vi "定点周期设置.vi"(11 "TimingControl 输入":refnum<class "TimingControl.lvclass">) -> (3 "TimingControl 输出":refnum<class "TimingControl.lvclass">)   [LabVIEW 2016, in "TimingControl.lvlib" / "TimingControl.lvclass"]
uses:
  TimingControl.lvclass
  TimingControl.lvclass/TimingControl.ctl
  <vilib>/Utility/miscctls.llb/LVPointTypeDef.ctl
panel:
  out "时间标识":timestamp format="%<%x %X>T"
  in  "每月启动":T1
  in  "每周启动":T2
  out "测试状态.结束时间":timestamp caption="结束时间" format="%<%y/%m/%d %H:%M:%S>T"
  out "测试状态.启动次数":dbl caption="启动次数"
  out "测试状态.启动时间":timestamp caption="启动时间" format="%<%y/%m/%d %H:%M:%S>T"
  in  "测量参数":T3 items=["氨氮"]
  in  "保存":bool
  in  "退出":bool
  in  "批量设置":bool
  out "周期模式选择卡":enum32{"选项卡 1", "选项卡 2"}(tab)
  in  "定点周期":T4
  in  "间隔启动":T6
  in  "周期模式":T7
  # "分钟"
  # "次"
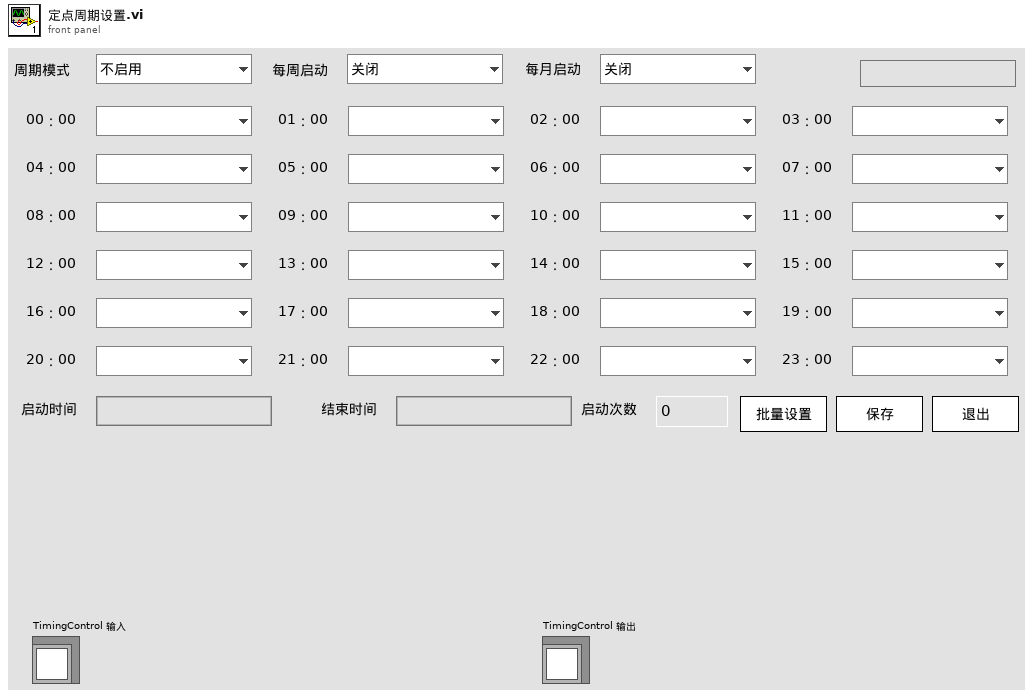
[diagram p1: front panel]
types:
  T1 = typedef "TimingControl.lvlib/TimingControl.lvclass/每月启动.ctl" = enum16{"关闭", "1号", "2号", "3号", "4号", "5号", "6号", "7号", "8号", "9号", "10号", "11号", "12号", "13号", "14号", "15号", "16号", "17号", "18号", "19号", "20号", "21号", "22号", "23号", "24号", "25号", "26号", "27号", "28号", "29号", "30号", "31号"}
  T2 = typedef "TimingControl.lvlib/TimingControl.lvclass/每周启动.ctl" = enum16{"关闭", "周日", "周一", "周二", "周三", "周四", "周五", "周六"}
  T3 = typedef "TimingControl.lvlib/TimingControl.lvclass/测量参数.ctl" = u16
  T4 = typedef "TimingControl.lvlib/TimingControl.lvclass/定点周期设置.ctl" = cluster{"启动命令":T5, "启动命令 2":T5, "启动命令 3":T5, "启动命令 4":T5, "启动命令 5":T5, "启动命令 6":T5, "启动命令 7":T5, "启动命令 8":T5, "启动命令 9":T5, "启动命令 10":T5, "启动命令 11":T5, "启动命令 12":T5, "启动命令 13":T5, "启动命令 14":T5, "启动命令 15":T5, "启动命令 16":T5, "启动命令 17":T5, "启动命令 18":T5, "启动命令 19":T5, "启动命令 20":T5, "启动命令 21":T5, "启动命令 22":T5, "启动命令 23":T5, "启动命令 24":T5}
  T5 = typedef "TimingControl.lvlib/TimingControl.lvclass/启动命令选择.ctl" = enum16{"", "水样测试", "标样核查", "零点核查", "跨度核查", "空白测试", "平行样测试", "加标回收", "空白校准", "标样校准", "初始化(清洗)"}
  T6 = typedef "TimingControl.lvlib/TimingControl.lvclass/间隔启动设置.ctl" = cluster{"启动命令":T5, "启动间隔":dbl, "启动次数":i32}
  T7 = typedef "TimingControl.lvlib/TimingControl.lvclass/周期模式设置.ctl" = enum16{"不启用", "定点模式", "间隔模式"}
  T8 = typedef "LVPointTypeDef.ctl" = cluster{"Horizontal":i16, "Vertical":i16}
  T9 = cluster{"启动时间":timestamp, "结束时间":timestamp, "启动次数":dbl}
  T10 = typedef "TimingControl.lvlib/TimingControl.lvclass/State Data.ctl" = cluster{"仪器时间":timestamp, "仪器运行状态":bool, "配置文件路径":path, "测量参数":u16, "测试状态":cluster{"启动时间":timestamp, "结束时间":timestamp, "启动次数":i32}, "配置信息":T11}
  T11 = typedef "TimingControl.lvlib/TimingControl.lvclass/配置信息.ctl" = cluster{"每周启动":T2, "每月启动":T1, "周期模式":T7, "测量参数":T3, "定点周期":T4, "间隔启动":T6, "配置时间":timestamp}
  T12 = cluster{"启动时间":timestamp, "结束时间":timestamp, "启动次数":i32}
  T13 = typedef "周期设置.lvlib/周期模式设置.ctl" = enum16{"不启用", "定点模式", "间隔模式"}
  T14 = typedef "LVDateTimeRec.ctl" = cluster{"秒数的小数部分":dbl, "秒":i32, "分":i32, "时":i32, "日":i32, "月":i32, "年":i32, "天数（周）":i32, "天数（年）":i32, "DST":i32}
  T15 = cluster{"每周启动":T2, "每月启动":T1, "周期模式":T7, "测量参数":T3, "定点周期":T4, cluster{"启动命令":T5, "启动间隔":dbl, "启动次数":i32}, "time stamp":timestamp}
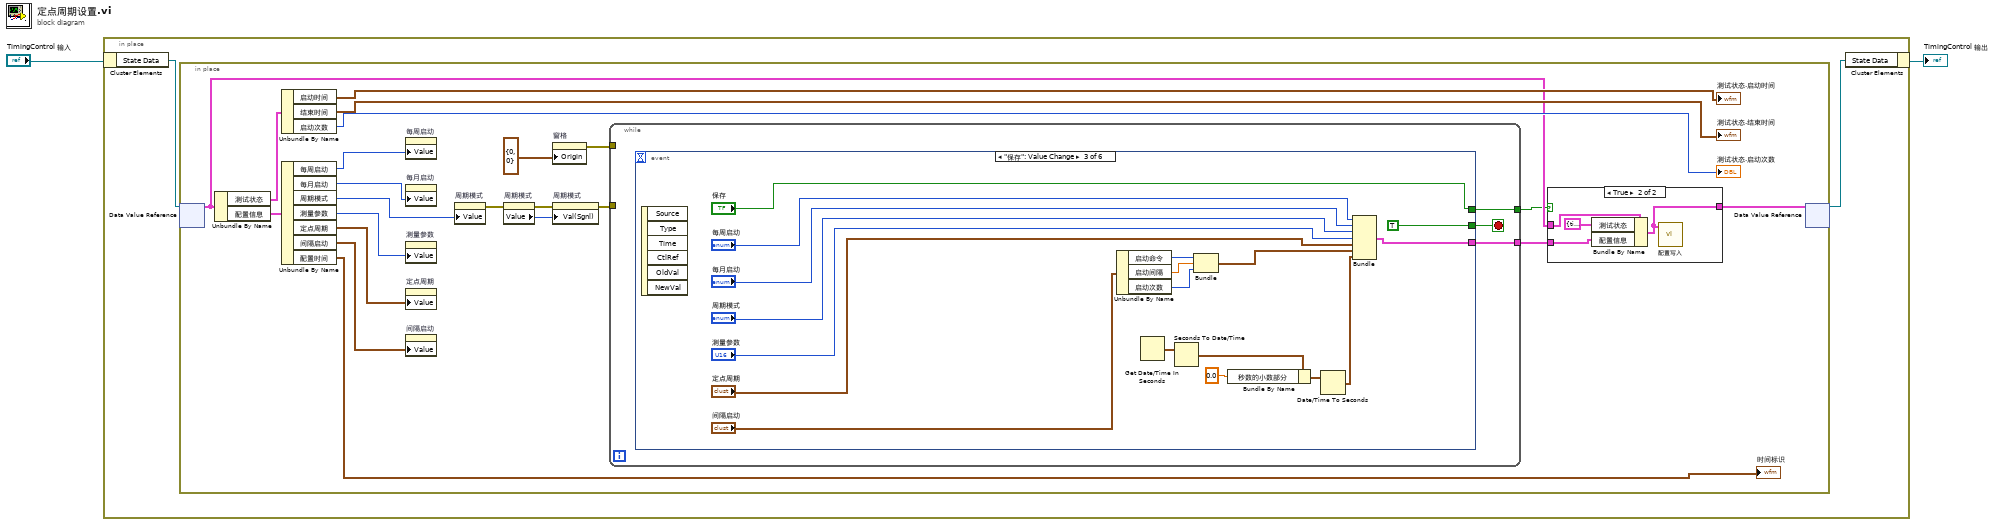
[diagram p0: block diagram]
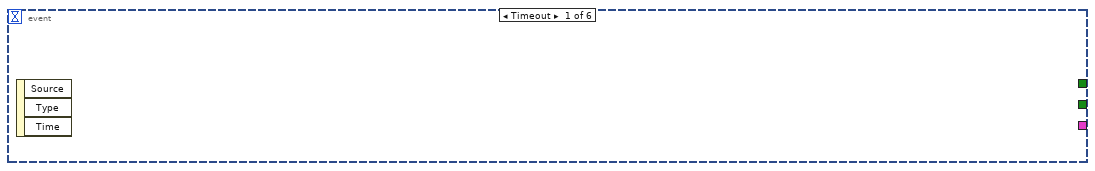
[diagram p3: hidden frame]
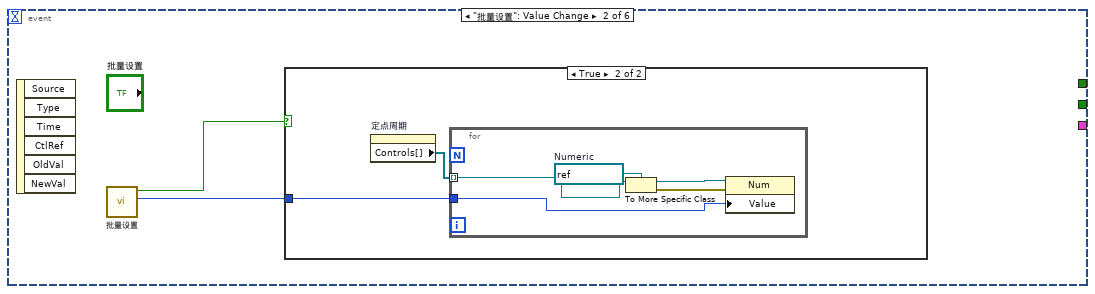
[diagram p4: hidden frame]
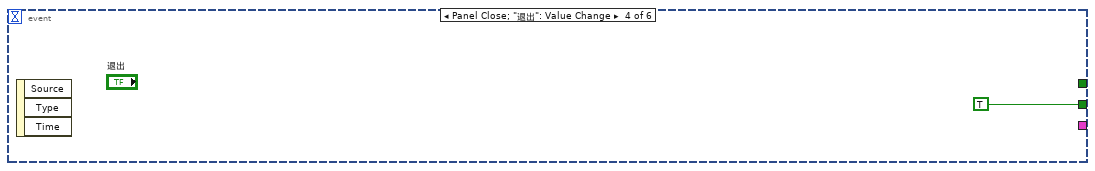
[diagram p6: hidden frame]
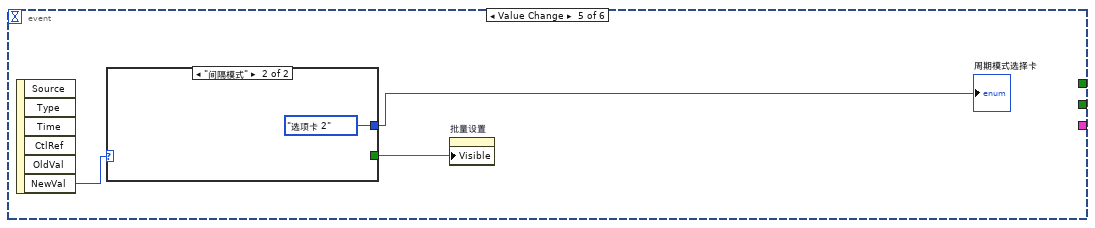
[diagram p7: hidden frame]
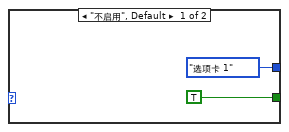
[diagram p8: hidden frame]
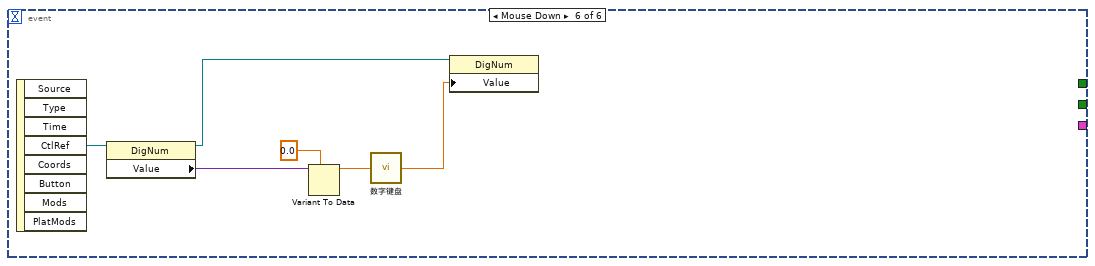
[diagram p9: hidden frame]
diagram:
  n1 = in-place {
    n2 = in-place-cluster #1("TimingControl 输入") -> ("State Data"=w4:refnum<data-value>)
    n3 = in-place {
      n4 = in-place-dvr #2(w4) -> (w9:T10)  [unwired: 1 out]
      n5 = Unbundle By Name(w9) -> ("测试状态"=w10:T12, "配置信息"=w11:T11)
      n6 = Unbundle By Name(w10) -> ("启动时间"=→"测试状态.启动时间":timestamp, "结束时间"=→"测试状态.结束时间":timestamp, "启动次数"=→"测试状态.启动次数":i32)
      n7 = Unbundle By Name(w11) -> ("每周启动"=w17:T2, "每月启动"=w16:T1, "周期模式"=w18:T7, "测量参数"=w15:T3, "定点周期"=w14:T4, "间隔启动"=w13:T6, "配置时间"=→"时间标识":timestamp)
      n8 = property on="每周启动" class="Enum (strict)"("Value"=w17) -> ()  [unwired: 2 in, 2 out]
      n9 = property on="每月启动" class="Enum (strict)"("Value"=w16) -> ()  [unwired: 2 in, 2 out]
      n10 = property on="测量参数" class="Ring (strict)"("Value"=w15) -> ()  [unwired: 2 in, 2 out]
      n11 = property on="定点周期" class="Clust (strict)"("Value"=w14) -> ()  [unwired: 2 in, 2 out]
      n12 = property on="间隔启动" class="Clust (strict)"("Value"=w13) -> ()  [unwired: 2 in, 2 out]
      n13 = property on="周期模式" class="Enum (strict)"("Value"=w18) -> (error out=w12:errorcluster)  [unwired: 2 in, 1 out]
      n14 = property on="周期模式" class="Enum (strict)"(error in=w12) -> (error out=w25:errorcluster, "Value"=w26:T13)  [unwired: 1 in, 1 out]
      n15 = property on="窗格" class="Pane"("Origin"=T8 {"Horizontal"=0, "Vertical"=0} ("原点")) -> (error out=w19:errorcluster)  [unwired: 2 in, 1 out]
      n16 = property on="周期模式" class="Enum (strict)"(error in=w25, "Val(Sgnl)"=w26) -> (error out=w24:errorcluster)  [unwired: 1 in, 1 out]
      n17 = while {
        tunnel: [w33] -> w7
        tunnel: w24 -> [_]
        tunnel: [w32] -> w6
        tunnel: w19 -> [_]
        stop <- w34 stop-if-true
        n18 = event shown="[2] \"保存\": Value Change" {
          selector: _ -> [_ _ _ _ _ _]
          dyn-events: _ -> [_ _ _ _ _ _]
          timeout: _ -> [_ _ _ _ _ _]
          tunnel: [_ _ TRUE TRUE _ _] -> w34
          tunnel: [_ _ w60 _ _ _] -> w33
          tunnel: [_ _ "保存" _ _ _] -> w32
          event Timeout {
            n19 = event-data() -> ()  [unwired: 1 in, 3 out]
          }
          event "批量设置": Value Change {
            n20 = event-data() -> ()  [unwired: 1 in, 6 out]
            n21 = call "批量设置.vi"() -> ("启动命令 2"=w36:T5, "确定 2"=w35:bool)  [unwired: 10 in]
            n22 = case shown="True" w35 {
              tunnel: w36 -> [_ w37]
              frame False {
              }
              frame True {
                n23 = property on="定点周期" class="Clust (strict)"() -> ("Controls[]"=w38:refnum<vi>[])  [unwired: 2 in, 2 out]
                n24 = for {
                  tunnel: w38 -> [w43] mode=indexing
                  tunnel: w37 -> [w39]
                  w42 = refnum<vi> refnum  # Numeric
                  n25 = To More Specific Class(target class=w42, reference=w43) -> (specific class reference=w41:refnum<vi>, error out=w40:errorcluster)  [unwired: 1 in]
                  n26 = property class="Num"(reference=w41, error in=w40, "Value"=w39) -> ()  [unwired: 2 out]
                }
              }
            }
          }
          event "保存": Value Change {
            n27 = event-data() -> ()  [unwired: 1 in, 6 out]
            n28 = Unbundle By Name("间隔启动") -> ("启动命令"=w57:T5, "启动间隔"=w56:dbl, "启动次数"=w55:i32)
            n29 = Get Date/Time In Seconds() -> (seconds since 1Jan1904=w47:timestamp)
            n30 = Seconds To Date/Time(time stamp (now)=w47) -> (date time rec=w46:T14)  [unwired: 1 in]
            n31 = Bundle("启动命令"=w57, "启动间隔"=w56, "启动次数"=w55) -> (w54:cluster{"启动命令":T5, "启动间隔":dbl, "启动次数":i32})  [unwired: 1 in]
            n32 = Bundle By Name(cluster=w46, "秒数的小数部分"=0.0) -> (w45:T14)
            n33 = Date/Time To Seconds(2:w45) -> (0:w48:timestamp)  [unwired: 1 in]
            n34 = Bundle("每周启动"="每周启动", "每月启动"="每月启动", "周期模式"="周期模式", "测量参数"="测量参数", "定点周期"="定点周期", w54, "time stamp"=w48) -> (w60:T15)  [unwired: 1 in]
          }
          event Panel Close; "退出": Value Change {
            n35 = event-data() -> ()  [unwired: 1 in, 3 out]
          }
          event Value Change {
            n36 = event-data() -> ("NewVal"=w64:T7)  [unwired: 1 in, 5 out]
            n37 = case shown="\"间隔模式\"" w64 {
              tunnel: [TRUE ("可见") _] -> w65
              tunnel: [enum32{"选项卡 1", "选项卡 2"}."选项卡 1" ("周期模式选择卡") enum32{"选项卡 1", "选项卡 2"}."选项卡 2" ("周期模式选择卡")] -> w63
              frame "不启用", Default {
              }
              frame "间隔模式" {
              }
            }
            "周期模式选择卡" <- w63
            n38 = property on="批量设置" class="Bool"("Visible"=w65) -> ()  [unwired: 2 in, 2 out]
          }
          event Mouse Down {
            n39 = event-data() -> ("CtlRef"=w74:refnum<vi>)  [unwired: 1 in, 7 out]
            n40 = property class="DigNum"(reference=w74) -> (reference out=w73:refnum<vi>, "Value"=w72:variant)  [unwired: 1 in, 1 out]
            n41 = Variant To Data(type=0.0, Variant=w72) -> (data=w70:dbl)  [unwired: 1 in, 1 out]
            n42 = call "数字键盘.vi"("OldNumber"=w70) -> ("NewNumber"=w69:sgl)
            n43 = property class="DigNum"(reference=w73, "Value"=w69) -> ()  [unwired: 1 in, 2 out]
          }
        }
      }
      n44 = case shown="True" w6 {
        tunnel: w9 -> [w27 w31]
        tunnel: [w27 w28] -> w8
        tunnel: w7 -> [_ w30]
        frame False {
        }
        frame True {
          n45 = Bundle By Name(cluster=w31, "测试状态"=T9 {"启动时间"=timestamp(0 s since 1904-01-01), "结束时间"=timestamp(0 s since 1904-01-01), "启动次数"=0.0}, "配置信息"=w30) -> (w28:T10)
          n46 = call "配置写入.vi"("数据值"=w28) -> ()  [unwired: 10 in, 1 out]
        }
      }
      n47 = in-place-dvr #2(w8) -> (w3:refnum<data-value>)  [unwired: 1 out]
    }
    n48 = in-place-cluster #1("State Data"=w3) -> (→"TimingControl 输出":refnum<class "TimingControl.lvclass">)
  }
